vi "observacao_queued.vi"() -> ()   [LabVIEW 2012, in "Shared_160.lvlib"] (continued)
                  tunnel: [TRUE FALSE] -> w2394
                  tunnel: [FALSE TRUE] -> w2393
                  frame False {
                  }
                  frame True {
                  }
                }
                "Recuar" <- w2394
                "Avancar" <- w2393
                n1886 = event shown="[1] \"Sent_EspDesvFeixe\": Value Change" {
                  selector: _ -> [_ _ _]
                  dyn-events: _ -> [_ _ _]
                  timeout: w2396 -> [_ _ _]
                  event Timeout {
                    n1887 = event-data() -> ()  [unwired: 1 in, 2 out]
                  }
                  event "Sent_EspDesvFeixe": Value Change {
                    n1888 = event-data() -> ()  [unwired: 1 in, 4 out]
                    n1889 = case shown="1" "Disabled" {
                      tunnel: ["RECUAR" ("Comando") "AVANCAR" ("Comando")] -> w2443
                      tunnel: ["ESP_LAMP" ("Dispositivo") "ESP_LAMP" ("Dispositivo")] -> w2442
                      frame 0, Default {
                        # "Case False (Default) em\noperação normal, com o\nbotão Sent_EspDesvFeixe\nligado ao ? deste case."
                      }
                      frame 1 {
                        # "CaseTrue. Cf. nota no case 0"
                        n1890 = property on="SlideCam1" class="Slide (strict)"("Visible"=TRUE) -> ()  [unwired: 2 in, 2 out]
                        n1891 = property on="stopCam1" class="Bool"("Visible"=FALSE) -> ()  [unwired: 2 in, 2 out]
                        "SlideCam1" <- u8 5 ("Slide 2")
                      }
                    }
                    n1892 = case shown="True" "Case Constant\n(See Context Help) 9" {
                      tunnel: w2443 -> [_ w2446]
                      tunnel: w2442 -> [_ w2445]
                      frame False {
                      }
                      frame True {
                        w2444 = u16 3 items=["ZERO", "AH", "DEC", "TUBO", "CUP"] ("Controlador")
                        n1893 = call "Monta Comando.vi"("Comando"=w2446, "Dispositivo"=w2445, "Controlador"=w2444) -> ()  [unwired: 4 in, 3 out]
                      }
                    }
                  }
                  event "Go_filtro": Value Change {
                    n1894 = event-data() -> ()  [unwired: 1 in, 6 out]
                    n1895 = case shown="True" "Go_filtro" {
                      frame False {
                      }
                      frame True {
                        (unwired) "ZERO: Porta serial da CAM1"
                        w2455 = u16 0 items=["ZERO", "AH", "DEC", "TUBO", "CUP"] ("Controlador")
                        n1896 = call "Monta Comando.vi"("Set Point"="Filtro", "Controlador"=w2455) -> ()  [unwired: 5 in, 3 out]
                      }
                    }
                  }
                }
                n1897 = case shown="False" "Velocidade" {
                  tunnel: [TRUE FALSE] -> w2391
                  tunnel: [FALSE TRUE] -> w2390
                  frame False {
                  }
                  frame True {
                  }
                }
                "Rapido" <- w2391
                "Lento" <- w2390
                n1898 = call "Bit Status TUBO.vi"("NomeStatus"=w2405) -> ("StatBit"=w2402:bool)
                n1899 = call "Bit Status TUBO.vi"("NomeStatus"=w2404) -> ("StatBit"=w2401:bool)
                n1900 = call "Bit Status TUBO.vi"("NomeStatus"=w2403) -> ("StatBit"=w2400:bool)
                n1901 = Not(x=w2402) -> (.not. x?=w2411:bool)
                n1902 = And(x=w2402, y=w2401) -> (x .and. y?=w2407:bool)
                "LedRepCam1" <- w2407
                n1903 = Or(x=w2401, y=w2400) -> (x .or. y?=w2412:bool)
                n1904 = And(x=w2402, y=w2400) -> (x .and. y?=w2406:bool)
                "LedCalCam1" <- w2406
                n1905 = property on="SlideCam1" class="Slide (strict)"() -> ("Visible"=w2409:bool)  [unwired: 2 in, 2 out]
                n1906 = Or(x=w2407, y=w2406) -> (x .or. y?=w2410:bool)
                n1907 = And(x=w2411, y=w2412) -> (x .and. y?=w2398:bool)
                n1908 = case shown="True" "Case Constant\n(See Context Help) 10" {
                  frame False {
                  }
                  frame True {
                    w2470 = FALSE
                    w2473 = u16 3 items=["ZERO", "AH", "DEC", "TUBO", "CUP"] ("Controlador")
                    w2471 = u8 0 ("Disabled")
                    n1909 = call "Monta Comando.vi"("Comando"="DESLIGAR", "Dispositivo"="ESP_LAMP", "Controlador"=w2473) -> ()  [unwired: 4 in, 3 out]
                    n1910 = property on="Sent_EspDesvFeixe" class="Bool (strict)"("Disabled"=w2471) -> ()  [unwired: 2 in, 2 out]
                    n1911 = property on="Go_filtro" class="Bool"("Disabled"=w2471) -> ()  [unwired: 2 in, 2 out]
                    n1912 = property on="stopCam1" class="Bool"("Visible"=w2470) -> ()  [unwired: 2 in, 2 out]
                    n1913 = property on="SlideCam1" class="Slide (strict)"("Visible"=w2470) -> ()  [unwired: 2 in, 2 out]
                  }
                }
                n1914 = And(x="Case Constant\n(See Context Help) 10", y=w2398) -> (x .and. y?=w2399:bool)
                n1915 = And(x=w2409, y=w2410) -> (x .and. y?=w2408:bool)
                n1916 = case shown="True" w2399 {
                  frame False {
                  }
                  frame True {
                    w2458 = u8 2 ("Disabled")
                    n1917 = local read "SlideCam1"() -> (w2457:u8)
                    n1918 = Add(x=w2457, y=u8 5) -> (x+y=w2459:u8)
                    n1919 = property on="Sent_EspDesvFeixe" class="Bool (strict)"("Disabled"=w2458) -> ()  [unwired: 2 in, 2 out]
                    n1920 = property on="Go_filtro" class="Bool"("Disabled"=w2458) -> ()  [unwired: 2 in, 2 out]
                    n1921 = Greater Or Equal?(x=w2459, y=u8 100 ("x")) -> (x >= y?=w2461:bool)
                    n1922 = case shown="True" w2461 {
                      selector: w2461 -> [_ w2465]
                      tunnel: w2459 -> [w2463 _]
                      frame False {
                        n1923 = local write "SlideCam1"(w2463) -> ()
                        n1924 = property on="SlideCam1" class="Slide (strict)"("Fill Color"=u32 16750950 ("color(black)")) -> ()  [unwired: 2 in, 2 out]
                      }
                      frame True {
                        n1925 = property on="stopCam1" class="Bool"("Visible"=w2465) -> ()  [unwired: 2 in, 2 out]
                        n1926 = local write "SlideCam1"(u8 90 ("Slide 2")) -> ()
                        n1927 = property on="SlideCam1" class="Slide (strict)"("Fill Color"=u32 16724787 ("color(black)")) -> ()  [unwired: 2 in, 2 out]
                      }
                    }
                  }
                }
                n1928 = case shown="True" w2408 {
                  frame False {
                  }
                  frame True {
                    w2469 = u8 0 ("Disabled")
                    n1929 = property on="Go_filtro" class="Bool"("Disabled"=w2469) -> ()  [unwired: 2 in, 2 out]
                    n1930 = property on="Sent_EspDesvFeixe" class="Bool (strict)"("Disabled"=w2469) -> ()  [unwired: 2 in, 2 out]
                    n1931 = property on="SlideCam1" class="Slide (strict)"("Visible"=FALSE) -> ()  [unwired: 2 in, 2 out]
                  }
                }
              }
              frame "Cam 2" {
                # "Cam 2"
              }
              frame "Cam IV." {
                # "Cam IV"
              }
              frame "Polarim." {
                # "Polarimetro"
              }
              frame "Fotrap" {
                # "Fotrap"
              }
              frame "Coude", Default {
                # "COUDE"
                n1932 = stacked-sequence {
                  frame #0 {
                    w2477 = u16 5 items=["Alarme", "Atencao", "Erro", "Ocupado", "Stop#3", "Cass#3", "MovFoco", "PosSecund", "Mov#2", "Mov#3", "Mov#4", "EspLamp", "HE", "NE", "EspLampRepouso", "EspLampCalibra"] ("NomeStatus")
                    w2476 = u16 7 items=["Alarme", "Atencao", "Erro", "Ocupado", "Stop#3", "Cass#3", "MovFoco", "PosSecund", "Mov#2", "Mov#3", "Mov#4", "EspLamp", "HE", "NE", "EspLampRepouso", "EspLampCalibra"] ("NomeStatus")
                    n1933 = local read "EspAtual"() -> (w2479:string)
                    n1934 = case shown="\"A\"" w2479 {
                      frame "X", Default {
                        w2480 = FALSE
                        n1935 = local write "ledVisivel"(w2480) -> ()
                        n1936 = local write "ledAzul"(w2480) -> ()
                        n1937 = local write "ledVermelho"(w2480) -> ()
                      }
                      frame "M" {
                        w2481 = FALSE
                        n1938 = local write "ledAzul"(w2481) -> ()
                        n1939 = local write "ledVermelho"(w2481) -> ()
                        n1940 = local write "ledVisivel"(w2481) -> ()
                      }
                      frame "A" {
                        # "Espelho A --> Azul\nEspelho B --> Visível\nEspelho C --> Vermelho"
                        n1941 = local write "ledVermelho"(FALSE) -> ()
                        n1942 = local write "ledVisivel"(FALSE) -> ()
                        n1943 = local write "ledAzul"(TRUE) -> ()
                      }
                      frame "B" {
                        # "Espelho A --> Azul\nEspelho B --> Visível\nEspelho C --> Vermelho"
                        n1944 = local write "ledVermelho"(FALSE) -> ()
                        n1945 = local write "ledVisivel"(TRUE) -> ()
                        n1946 = local write "ledAzul"(FALSE) -> ()
                      }
                      frame "C" {
                        # "Espelho A --> Azul\nEspelho B --> Visível\nEspelho C --> Vermelho"
                        n1947 = local write "ledVermelho"(TRUE) -> ()
                        n1948 = local write "ledVisivel"(FALSE) -> ()
                        n1949 = local write "ledAzul"(FALSE) -> ()
                      }
                    }
                    n1950 = call "Bit Status TUBO.vi"("NomeStatus"=w2477) -> ("StatBit"=→"Cjto_3":bool)
                    n1951 = call "Bit Status TUBO.vi"("NomeStatus"=w2476) -> ("StatBit"=→"PosSecundario":bool)
                  }
                  frame #1 {
                    w2501 = u16 5 items=["Alarme", "Atencao", "Erro", "Ocupado", "Stop#3", "Cass#3", "MovFoco", "PosSecund", "Mov#2", "Mov#3", "Mov#4", "EspLamp", "HE", "NE", "EspLampRepouso", "EspLampCalibra"] ("NomeStatus")
                    w2506 = u16 8 items=["Alarme", "Atencao", "Erro", "Ocupado", "Stop#3", "Cass#3", "MovFoco", "PosSecund", "Mov#2", "Mov#3", "Mov#4", "EspLamp", "HE", "NE", "EspLampRepouso", "EspLampCalibra"] ("NomeStatus")
                    w2507 = u16 9 items=["Alarme", "Atencao", "Erro", "Ocupado", "Stop#3", "Cass#3", "MovFoco", "PosSecund", "Mov#2", "Mov#3", "Mov#4", "EspLamp", "HE", "NE", "EspLampRepouso", "EspLampCalibra"] ("NomeStatus")
                    w2508 = u16 10 items=["Alarme", "Atencao", "Erro", "Ocupado", "Stop#3", "Cass#3", "MovFoco", "PosSecund", "Mov#2", "Mov#3", "Mov#4", "EspLamp", "HE", "NE", "EspLampRepouso", "EspLampCalibra"] ("NomeStatus")
                    w2519 = u16 4 items=["Alarme", "Atencao", "Erro", "Ocupado", "Stop#3", "Cass#3", "MovFoco", "PosSecund", "Mov#2", "Mov#3", "Mov#4", "EspLamp", "HE", "NE", "EspLampRepouso", "EspLampCalibra"] ("NomeStatus")
                    w2520 = u16 3 items=["Alarme", "Atencao", "Erro", "Ocupado", "Stop#3", "Cass#3", "MovFoco", "PosSecund", "Mov#2", "Mov#3", "Mov#4", "EspLamp", "HE", "NE", "EspLampRepouso", "EspLampCalibra"] ("NomeStatus")
                    # "CJTO#3 EM \nMOVIMENTO"
                    n1952 = local read "PosSecundario"() -> (w2499:bool)
                    n1953 = call "Bit Status TUBO.vi"("NomeStatus"=w2520) -> ("StatBit"=w2495:bool)
                    n1954 = call "Bit Status TUBO.vi"("NomeStatus"=w2506) -> ("StatBit"=w2512:bool)
                    "#2" <- w2512
                    n1955 = call "Bit Status TUBO.vi"("NomeStatus"=w2507) -> ("StatBit"=w2511:bool)
                    "#3" <- w2511
                    n1956 = call "Bit Status TUBO.vi"("NomeStatus"=w2508) -> ("StatBit"=w2510:bool)
                    "#4" <- w2510
                    n1957 = call "Bit Status TUBO.vi"("NomeStatus"=w2501) -> ("StatBit"=w2498:bool)
                    n1958 = call "Bit Status TUBO.vi"("NomeStatus"=w2519) -> ("StatBit"=w2497:bool)
                    n1959 = Not Equal?(x=w2499, y=w2498) -> (x != y?=w2500:bool)
                    n1960 = Not(x=w2497) -> (.not. x?=w2493:bool)
                    n1961 = And(x=w2500, y=w2497) -> (x .and. y?=w2494:bool)
                    n1962 = Compound Arithmetic op=OR(w2512, w2511, w2510) -> (w2509:bool)
                    n1963 = Compound Arithmetic op=OR(w2494, w2493, w2495) -> (w2496:bool)
                    n1964 = property on="PosSecundario" class="Bool (strict)"("Blinking"=w2494) -> ()  [unwired: 2 in, 2 out]
                    n1965 = property on="Cjto_3" class="Bool (strict)"("Blinking"=w2494) -> ()  [unwired: 2 in, 2 out]
                    n1966 = case shown="True" w2496 {
                      tunnel: [T6."Page Enabled" ("Page Enabled State") T6."Page Disabled" ("Page Enabled State")] -> w2491
                      tunnel: [u8 0 ("Disabled") u8 2 ("Disabled")] -> w2505
                      frame False {
                      }
                      frame True {
                      }
                    }
                    n1967 = property on="MENSAGEM" class="Str"("Visible"=w2493, "Blinking"=w2493) -> ()  [unwired: 2 in, 2 out]
                    n1968 = case shown="True" w2509 {
                      tunnel: w2505 -> [w2524 _]
                      tunnel: [w2524 u8 2 ("Disabled")] -> w2504
                      tunnel: [FALSE TRUE] -> w2503
                      tunnel: [FALSE ("Blinking") TRUE ("Blinking")] -> w2502
                      frame False {
                        n1969 = local write "MENSAGEM 2"("EM MOVIMENTO" ("MENSAGEM 2")) -> ()
                      }
                      frame True {
                        n1970 = local read "EndTime"() -> (w2533:u32)
                        n1971 = Tick Count (ms)() -> (millisecond timer value=w2532:u32)
                        n1972 = Subtract(x=w2533, y=w2532) -> (x-y=w2531:u32)
                        n1973 = Divide(x=w2531, y=u32 1000) -> (x/y=w2528:dbl)
                        n1974 = To Unsigned Long Integer(number=w2528) -> (unsigned 32bit integer=w2529:u32)
                        n1975 = Number To Decimal String(number=w2529) -> (decimal integer string=w2526:string)  [unwired: 1 in]
                        n1976 = Concatenate Strings("EM MOVIMENTO " ("MENSAGEM 2"), w2526) -> (w2527:string)
                        n1977 = local write "MENSAGEM 2"(w2527) -> ()
                      }
                    }
                    n1978 = property on="Setup, Pointing & Guiding" class="TabCtl (strict)"() -> ("Pages"=w2492:refnum<vi>[])  [unwired: 2 in, 2 out]
                    n1979 = Index Array(array=w2492, index=4) -> (element=w2515:refnum<vi>)
                    n1980 = Index Array(array=w2492, index=5) -> (element=w2518:refnum<vi>)
                    n1981 = property class="Page"(reference=w2515, "Page Enabled State"=w2491) -> ()  [unwired: 1 in, 2 out]
                    n1982 = property class="Page"(reference=w2518, "Page Enabled State"=w2491) -> ()  [unwired: 1 in, 2 out]
                    n1983 = case shown="False" w2499 {
                      tunnel: [u8 0 ("Disabled") w2539] -> w2514
                      tunnel: w2504 -> [w2537 _]
                      tunnel: [w2537 w2539] -> w2513
                      frame False {
                        # "COUDE"
                      }
                      frame True {
                        w2539 = u8 2 ("Disabled")
                        # "CASS"
                      }
                    }
                    n1984 = property on="MENSAGEM 2" class="Str"("Visible"=w2503, "Blinking"=w2502) -> ()  [unwired: 2 in, 2 out]
                    n1985 = property on="ledAzul" class="Bool (strict)"("Disabled"=w2514) -> ()  [unwired: 2 in, 2 out]
                    n1986 = property on="ledVisivel" class="Bool (strict)"("Disabled"=w2514) -> ()  [unwired: 2 in, 2 out]
                    n1987 = property on="ledVermelho" class="Bool (strict)"("Disabled"=w2514) -> ()  [unwired: 2 in, 2 out]
                    n1988 = property on="Radio Buttons" class="RadioBtnsControl (strict)"("Disabled"=w2514) -> ()  [unwired: 2 in, 2 out]
                    n1989 = property on="#2" class="Bool (strict)"("Disabled"=w2514) -> ()  [unwired: 2 in, 2 out]
                    n1990 = property on="#3" class="Bool (strict)"("Disabled"=w2514) -> ()  [unwired: 2 in, 2 out]
                    n1991 = property on="#4" class="Bool (strict)"("Disabled"=w2514) -> ()  [unwired: 2 in, 2 out]
                    n1992 = property on="Go_Coudé" class="Bool"("Disabled"=w2513) -> ()  [unwired: 2 in, 2 out]
                  }
                  frame #2 {
                    n1993 = case shown="False" "Go_Coudé" {
                      frame False {
                        w2545 = u16 2 items=["Alarme", "Atencao", "Erro", "Ocupado", "Stop#3", "Cass#3", "MovFoco", "PosSecund", "Mov#2", "Mov#3", "Mov#4", "EspLamp", "HE", "NE", "EspLampRepouso", "EspLampCalibra"] ("NomeStatus")
                        w2546 = u16 3 items=["Alarme", "Atencao", "Erro", "Ocupado", "Stop#3", "Cass#3", "MovFoco", "PosSecund", "Mov#2", "Mov#3", "Mov#4", "EspLamp", "HE", "NE", "EspLampRepouso", "EspLampCalibra"] ("NomeStatus")
                        # "TRATA ERROS DO CONTROLADOR"
                        n1994 = call "Bit Status TUBO.vi"("NomeStatus"=w2545) -> ("StatBit"=w2548:bool)
                        n1995 = call "Bit Status TUBO.vi"("NomeStatus"=w2546) -> ("StatBit"=w2550:bool)
                        n1996 = Not(x=w2550) -> (.not. x?=w2549:bool)
                        n1997 = And(x=w2548, y=w2549) -> (x .and. y?=w2547:bool)
                        n1998 = case shown="True" w2547 {
                          frame False {
                          }
                          frame True {
                            w2553 = u16 3 items=["ZERO", "AH", "DEC", "TUBO", "CUP"] ("Controlador")
                            n1999 = call "Monta Comando.vi"("Comando"="ERROS", "Dispositivo"="PROG" ("Comando"), "Controlador"=w2553) -> ()  [unwired: 4 in, 3 out]
                          }
                        }
                      }
                      frame True {
                        w2554 = u16 3 items=["ZERO", "AH", "DEC", "TUBO", "CUP"] ("Controlador")
                        # "Enviar comando de \nmudar Espelho ABC"
                        n2000 = local read "EspAtual"() -> (w2560:string)
                        n2001 = case shown="\"Visível\"" "Radio Buttons" {
                          tunnel: ["C" ("Comando") "A" ("Comando") "B" ("Comando")] -> w2555
                          tunnel: w2560 -> [w2563 w2569 w2574]
                          tunnel: [w2562 w2568 w2575] -> w2557
                          frame "Vermelho" {
                            n2002 = case shown="\"A\"" w2563 {
                              tunnel: [u32 0 u32 60000 u32 35000] -> w2562
                              frame "C", Default {
                              }
                              frame "B" {
                              }
                              frame "A" {
                              }
                            }
                          }
                          frame "Azul", Default {
                            n2003 = case shown="\"C\"" w2569 {
                              tunnel: [u32 0 u32 35000 u32 60000] -> w2568
                              frame "A", Default {
                              }
                              frame "B" {
                              }
                              frame "C" {
                              }
                            }
                          }
                          frame "Visível" {
                            n2004 = case shown="\"C\"" w2574 {
                              tunnel: [u32 0 u32 60000 u32 35000] -> w2575
                              frame "B", Default {
                              }
                              frame "A" {
                              }
                              frame "C" {
                              }
                            }
                          }
                        }
                        n2005 = Tick Count (ms)() -> (millisecond timer value=w2559:u32)
                        n2006 = Add(x=w2559, y=w2557) -> (x+y=→"EndTime":u32)
                        n2007 = call "Monta Comando.vi"("Comando"=w2555, "Dispositivo"="ESPELHO" ("Comando"), "Controlador"=w2554) -> ()  [unwired: 4 in, 3 out]
                      }
                    }
                  }
                  frame #3 {
                    w2586 = 360.0
                    w2591 = 6.283185307179586
                    n2008 = global read "Global_Telescopio.vi" "guide_ang"() -> (w2601:string)
                    n2009 = global read "Global_Telescopio.vi" "guide_nor"() -> (w2602:string)
                    n2010 = global read "Global_Telescopio.vi" "AH_now"() -> (w2598:dbl)
                    n2011 = global read "Global_Telescopio.vi" "delta_now"() -> (w2599:dbl)
                    n2012 = Add(x=w2598, y=w2599) -> (x+y=w2590:dbl)
                    n2013 = Fract/Exp String To Number(string=w2601) -> (number=w2597:dbl)  [unwired: 3 in, 1 out]
                    n2014 = Fract/Exp String To Number(string=w2602) -> (number=w2600:dbl)  [unwired: 3 in, 1 out]
                    n2015 = Quotient & Remainder(x=w2590, y=w2591) -> (x-y*floor(x/y)=w2593:dbl)  [unwired: 1 out]
                    n2016 = Add(x=w2597, y=w2600) -> (x+y=w2582:dbl)
                    n2017 = Less Than 0?(x=w2593) -> (x < 0?=w2595:bool)
                    n2018 = case shown="True" w2595 {
                      tunnel: w2593 -> [w2603 w2606]
                      tunnel: [w2603 w2604] -> w2592
                      tunnel: w2591 -> [_ w2605]
                      frame False {
                      }
                      frame True {
                        n2019 = Add(x=w2606, y=w2605) -> (x+y=w2604:dbl)
                      }
                    }
                    n2020 = Add(x=124.0, y=w2582) -> (x+y=w2581:dbl)
                    n2021 = Multiply(x=w2592, y=57.29577951 ("x*y")) -> (x*y=w2589:dbl)
                    n2022 = Subtract(x=98.2, y=w2589) -> (x-y=w2588:dbl)
                    n2023 = Add(x=w2581, y=w2588) -> (x+y=w2585:dbl)
                    n2024 = Quotient & Remainder(x=w2585, y=w2586) -> (floor(x/y)=w2587:dbl)  [unwired: 1 out]
                    n2025 = Multiply(x=w2587, y=w2586) -> (x*y=w2584:dbl)
                    n2026 = Subtract(x=w2585, y=w2584) -> (x-y=→"Ang. Fenda":dbl)
                  }
                  frame #4 {
                    # "90"
                    # "270"
                    # "180"
                    # "0"
                    n2027 = event shown="[0] Timeout" {
                      selector: _ -> [_ _ _ _ _ _ _ _ _ _ _]
                      dyn-events: _ -> [_ _ _ _ _ _ _ _ _ _ _]
                      timeout: 10 -> [_ _ _ _ _ _ _ _ _ _ _]
                      event Timeout {
                        n2028 = event-data() -> ()  [unwired: 1 in, 2 out]
                        n2029 = stacked-sequence {
                          frame #0 {
                            n2030 = local read "parou 3"() -> (w2608:bool)
                            n2031 = case shown="True" w2608 {
                              frame False {
                              }
                              frame True {
                                n2032 = call "InstrumentControl.vi"("Input Message"="COUDE REDE POSICAO") -> ("Output Message"=w2611:string)  [unwired: 9 in, 1 out]
                                "Output Message" <- w2611
                                n2033 = Decimal String To Number(string=w2611) -> (number=w2610:i32)  [unwired: 2 in, 1 out]
                                n2034 = while {
                                shift-right: [w2614] -> w2609
                                shift-left: _ -> [w2618]
                                tunnel: w2610 -> [w2614]
                                stop <- TRUE stop-if-true
                                n2035 = Subtract(x=w2618, y=w2614) -> (x-y=w2617:i32)
                                n2036 = Absolute Value(x=w2617) -> (abs(x)=w2616:i32)
                                n2037 = Greater Or Equal?(x=w2616, y=1) -> (x >= y?=→"parou 3":bool)
                                }
                                "Posição Rede" <- w2609
                              }
                            }
                          }
                          frame #1 {
                            n2038 = local read "parou"() -> (w2621:bool)
                            n2039 = local read "parou 2"() -> (w2620:bool)
                            n2040 = case shown="True" w2620 {
                              frame False {
                              }
                              frame True {
                                # "Cada volta -> 10mm\nCada volta -> 4000counts\n1 count = 0,0025mm"
                                n2041 = call "InstrumentControl.vi"("Input Message"="COUDE ESPELHO POSICAO") -> ("Output Message"=w2628:string)  [unwired: 9 in, 1 out]
                                n2042 = Fract/Exp String To Number(string=w2628) -> (number=w2627:dbl)  [unwired: 3 in, 1 out]
                                n2043 = while {
                                shift-right: [w2640] -> w2623
                                shift-left: _ -> [w2641]
                                tunnel: w2627 -> [w2640]
                                tunnel: [w2636] -> w2622
                                stop <- TRUE stop-if-true
                                n2044 = Subtract(x=w2641, y=w2640) -> (x-y=w2639:dbl)
                                n2045 = Absolute Value(x=w2639) -> (abs(x)=w2638:dbl)
                                n2046 = Greater Or Equal?(x=w2638, y=0.02) -> (x >= y?=w2636:bool)
                                "parou 2" <- w2636
                                }
                                "Posição Espelho" <- w2623
                                n2047 = case shown="False" w2622 {
                                frame False {
                                n2048 = call "InstrumentControl.vi"("Input Message"="COUDE SERIAL CHAVEAR OFF") -> ()  [unwired: 9 in, 2 out]
                                }
                                frame True {
                                }
                                }
                                n2049 = Absolute Value(x=w2623) -> (abs(x)=w2624:dbl)
                                n2050 = Less Or Equal?(x=w2624, y=0.5) -> (x <= y?=w2626:bool)
                                n2051 = case shown="False" w2626 {
                                tunnel: w2624 -> [w2633 _]
                                frame False {
                                n2052 = Greater Or Equal?(x=w2633, y=34.5) -> (x >= y?=w2631:bool)
                                n2053 = case shown="True" w2631 {
                                frame False {
                                }
                                frame True {
                                n2054 = local write "Boolean"(TRUE ("Boolean")) -> ()
                                }
                                }
                                }
                                frame True {
                                n2055 = local write "Boolean"(FALSE ("Boolean")) -> ()
                                }
                                }
                              }
                            }
                            n2056 = case shown="True" w2621 {
                              frame False {
                              }
                              frame True {
                                n2057 = call "InstrumentControl.vi"("Input Message"="COUDE FENDA POSICAO") -> ("Output Message"=w2648:string)  [unwired: 9 in, 1 out]
                                n2058 = Fract/Exp String To Number(string=w2648) -> (number=w2647:dbl)  [unwired: 3 in, 1 out]
                                n2059 = Multiply(x=w2647, y=1000.0) -> (x*y=w2645:dbl)
                                n2060 = while {
                                shift-right: [w2655] -> w2644
                                shift-left: _ -> [w2656]
                                tunnel: w2645 -> [w2655]
                                tunnel: [w2651] -> w2643
                                stop <- TRUE stop-if-true
                                n2061 = Subtract(x=w2656, y=w2655) -> (x-y=w2654:dbl)
                                n2062 = Absolute Value(x=w2654) -> (abs(x)=w2653:dbl)
                                n2063 = Greater Or Equal?(x=w2653, y=1.0) -> (x >= y?=w2651:bool)
                                "parou" <- w2651
                                }
                                "Largura da Fenda 2" <- w2644
                                n2064 = case shown="False" w2643 {
                                frame False {
                                n2065 = call "InstrumentControl.vi"("Input Message"="COUDE SERIAL CHAVEAR OFF") -> ()  [unwired: 9 in, 2 out]
                                }
                                frame True {
                                }
                                }
                              }
                            }
                          }
                        }
                      }
                      event "Cathode": Value Change {
                        n2066 = event-data() -> ("NewVal"=w2658:bool)  [unwired: 1 in, 4 out]
                        n2067 = case shown="True" w2658 {
                          frame False {
                          }
                          frame True {
                            n2068 = flat-sequence {
                              frame #0 {
                                w2660 = FALSE ("NeAr")
                                n2069 = local write "Neon"(w2660) -> ()
                                n2070 = local write "Incand"(w2660) -> ()
                                n2071 = local write "Position"("Moving" ("Prisma Position")) -> ()
                                n2072 = call "Comando_Quick_Silver.vi"("COMANDO COMPLETO"="COUDE PRISMA MOVER 0" ("Input Message")) -> ()  [unwired: 2 in, 3 out]
                                n2073 = local write "IronArc"(w2660) -> ()
                              }
                              frame #1 {
                                n2074 = Wait (ms)(milliseconds to wait=u32 50) -> ()  [unwired: 1 out]
                              }
                              frame #2 {
                                n2075 = local write "Position"("Cathode" ("Prisma Position")) -> ()
                              }
                            }
                          }
                        }
                      }
                      event "Neon": Value Change {
                        n2076 = event-data() -> ("NewVal"=w2664:bool)  [unwired: 1 in, 4 out]
                        n2077 = case shown="True" w2664 {
                          frame False {
                          }
                          frame True {
                            n2078 = flat-sequence {
                              frame #0 {
                                w2666 = FALSE ("ThAr")
                                n2079 = local write "Cathode"(w2666) -> ()
                                n2080 = local write "Incand"(w2666) -> ()
                                n2081 = local write "Position"("Moving" ("Prisma Position")) -> ()
                                n2082 = call "Comando_Quick_Silver.vi"("COMANDO COMPLETO"="COUDE PRISMA MOVER 180" ("Input Message")) -> ()  [unwired: 2 in, 3 out]
                                n2083 = local write "IronArc"(w2666) -> ()
                              }
                              frame #1 {
                                n2084 = Wait (ms)(milliseconds to wait=u32 50) -> ()  [unwired: 1 out]
                              }
                              frame #2 {
                                n2085 = local write "Position"("Neon" ("Prisma Position")) -> ()
                              }
                            }
                          }
                        }
                      }
                      event "Incand": Value Change {
                        n2086 = event-data() -> ("NewVal"=w2670:bool)  [unwired: 1 in, 4 out]
                        n2087 = case shown="True" w2670 {
                          frame False {
                          }
                          frame True {
                            n2088 = flat-sequence {
                              frame #0 {
                                w2672 = FALSE ("ThAr")
                                n2089 = local write "Cathode"(w2672) -> ()
                                n2090 = local write "Neon"(w2672) -> ()
                                n2091 = local write "Position"("Moving" ("Prisma Position")) -> ()
                                n2092 = call "Comando_Quick_Silver.vi"("COMANDO COMPLETO"="COUDE PRISMA MOVER 270 " ("Input Message")) -> ()  [unwired: 2 in, 3 out]
                                n2093 = local write "IronArc"(w2672) -> ()
                              }
                              frame #1 {
                                n2094 = Wait (ms)(milliseconds to wait=u32 50) -> ()  [unwired: 1 out]
                              }
                              frame #2 {
                                n2095 = local write "Position"("Incand" ("Prisma Position")) -> ()
                              }
                            }
                          }
                        }
                      }
                      event Value Change {
                        n2096 = event-data() -> ("NewVal"=w2676:T4)  [unwired: 1 in, 4 out]
                        n2097 = case shown="True" w2676 {
                          frame False {
                          }
                          frame True {
                            n2098 = call "InstrumentControl.vi"("Input Message"="COUDE FENDA INICIAR") -> ()  [unwired: 9 in, 2 out]
                          }
                        }
                      }
                      event Value Change {
                        n2099 = event-data() -> ("NewVal"=w2678:T4)  [unwired: 1 in, 4 out]
                        n2100 = case shown="True" w2678 {
                          frame False {
                          }
                          frame True {
                            n2101 = call "Comando_Quick_Silver.vi"("COMANDO COMPLETO"="COUDE ESPELHO INICIAR" ("Input Message")) -> ()  [unwired: 2 in, 3 out]
                          }
                        }
                      }
                      event Value Change {
                        n2102 = event-data() -> ("NewVal"=w2680:T4)  [unwired: 1 in, 4 out]
                        n2103 = case shown="True" w2680 {
                          frame False {
                          }
                          frame True {
                            n2104 = call "InstrumentControl.vi"("Input Message"="COUDE PRISMA INICIAR") -> ()  [unwired: 9 in, 2 out]
                          }
                        }
                      }
                      event "Go Angulo de Difração": Value Change {
                        n2105 = event-data() -> ("NewVal"=w2682:bool)  [unwired: 1 in, 4 out]
                        n2106 = case shown="True" w2682 {
                          frame False {
                          }
                          frame True {
                            # "Envia comando para rede de difração"
                            n2107 = Number To Decimal String(number="Angulo da rede de difração") -> (decimal integer string=w2684:string)  [unwired: 1 in]
                            n2108 = Concatenate Strings("COUDE REDE MOVER ", w2684) -> (w2687:string)
                            n2109 = call "InstrumentControl.vi"("Input Message"=w2687) -> ()  [unwired: 9 in, 2 out]
                            n2110 = local write "parou 3"(TRUE ("parou 3")) -> ()
                          }
                        }
                      }
                      event "Go Largura da Fenda": Value Change {
                        n2111 = event-data() -> ("NewVal"=w2688:bool)  [unwired: 1 in, 4 out]
                        n2112 = case shown="True" w2688 {
                          frame False {
                          }
                          frame True {
                            n2113 = call "InstrumentControl.vi"("Input Message"="COUDE SERIAL CHAVEAR ON") -> ("error out"=w2690:errorcluster)  [unwired: 9 in, 1 out]
                            n2114 = Divide(x="Largura da Fenda", y=1000.0) -> (x/y=w2698:dbl)
                            n2115 = Number To Fractional String(use system decimal point (T)=FALSE, number=w2698, precision (6)=i16 6) -> (F-format string=w2692:string)  [unwired: 1 in]
                            n2116 = Concatenate Strings("COUDE FENDA MOVER ", w2692) -> (w2694:string)
                            n2117 = local write "parou"(TRUE ("parou")) -> ()
                            n2118 = call "InstrumentControl.vi"("error"=w2690, "Input Message"=w2694) -> ()  [unwired: 8 in, 2 out]
                          }
                        }
                      }
                      event "Prisma das Lâmpadas": Value Change {
                        n2119 = event-data() -> ("NewVal"=w2709:bool)  [unwired: 1 in, 4 out]
                        n2120 = case shown="False" w2709 {
                          tunnel: [0.0 ("y") 35.0 ("y")] -> w2707
                          frame False {
                            n2121 = local write "Boolean"(TRUE ("Boolean")) -> ()
                          }
                          frame True {
                            n2122 = local write "Boolean"(FALSE ("Boolean 2")) -> ()
                          }
                        }
                        n2123 = call "InstrumentControl.vi"("Input Message"="COUDE SERIAL CHAVEAR ON") -> ("error out"=w2701:errorcluster)  [unwired: 9 in, 1 out]
                        n2124 = local write "parou 2"(TRUE ("parou 2")) -> ()
                        n2125 = Number To Fractional String(use system decimal point (T)=FALSE, number=w2707, precision (6)=i16 6) -> (F-format string=w2702:string)  [unwired: 1 in]
                        n2126 = Concatenate Strings("COUDE ESPELHO MOVER ", w2702) -> (w2704:string)
                        n2127 = call "InstrumentControl.vi"("error"=w2701, "Input Message"=w2704) -> ()  [unwired: 8 in, 2 out]
                      }
                      event "IronArc": Value Change {
                        n2128 = event-data() -> ("NewVal"=w2714:bool)  [unwired: 1 in, 4 out]
                        n2129 = case shown="True" w2714 {
                          frame False {
                          }
                          frame True {
                            n2130 = flat-sequence {
                              frame #0 {
                                w2716 = FALSE ("ThAr")
                                n2131 = local write "Cathode"(w2716) -> ()
                                n2132 = local write "Neon"(w2716) -> ()
                                n2133 = local write "Position"("Moving" ("Prisma Position")) -> ()
                                n2134 = call "Comando_Quick_Silver.vi"("COMANDO COMPLETO"="COUDE PRISMA MOVER 90 " ("Input Message")) -> ()  [unwired: 2 in, 3 out]
                                n2135 = local write "Incand"(w2716) -> ()
                              }
                              frame #1 {
                                n2136 = Wait (ms)(milliseconds to wait=u32 50) -> ()  [unwired: 1 out]
                              }
                              frame #2 {
                                n2137 = local write "Position"("IronArc" ("Prisma Position")) -> ()
                              }
                            }
                          }
                        }
                      }
                    }
                  }
                }
              }
            }
          }
          frame "FOCUS" {
            w2743 = cluster{u32, u32}[] [] ("Colors [4]")
            w2744 = cluster{u32, u32}[] [] ("Colors [4]")
            # "ATUALIZA FOCO COM VALORES\nPUBLICADOS PELO FOCUSER160"
            # "dark(0)/bright(1)\n green"
            # "red(0)/greem(1)"
            # "ZeroMQ"
            # "T:  0x54      84\nC: 0x43       51\nS:  0x53      83\nP:  0x50      80\nD:  0x44      52\nClientId= 350"
            n2138 = global read "Global_Telescopio.vi" "queueSUB"() -> (w2738:refnum<queue>)
            n2139 = global read "Global_Telescopio.vi" "Focuser160"() -> (w2734:T11)
            n2140 = Get Queue Status(queue=w2738) -> (queue out=w2735:refnum<queue>, # elements in queue=w2737:i32)  [unwired: 2 in, 6 out]
            n2141 = Greater Than 0?(x=w2737) -> (x > 0?=w2736:bool)
            n2142 = call "TX focus FOCO.vi"("Comando"="pos") -> ("pos (deg)"=→"old":dbl)  [unwired: 12 in, 2 out]
            n2143 = case shown="True" w2736 {
              tunnel: w2735 -> [_ w2794]
              tunnel: w2734 -> [w2785 w2792]
              tunnel: [w2785 w2791] -> w2733
              frame False {
              }
              frame True {
                n2144 = Flush Queue(queue=w2794) -> (remaining elements=w2788:string[], error out=w2793:errorcluster)  [unwired: 1 in, 1 out]
                n2145 = Array Size(array=w2788) -> (size(s)=w2790:i32)
                "size(s)" <- w2790
                n2146 = Decrement(x=w2790) -> (x-1=w2789:i32)
                n2147 = Index Array(array=w2788, index=w2789) -> (element=w2787:string)
                "element" <- w2787
                n2148 = call "Focuser JSON to cluster.vi"("JSON status"=w2787) -> ("Focuser160"=w2786:T11)  [unwired: 10 in]
                n2149 = Select(t=w2792, s=w2793, f=w2786) -> (s? t:f=w2791:T11)
                n2150 = global write "Global_Telescopio.vi" "Focuser160"(w2791) -> ()
              }
            }
            n2151 = Unbundle By Name(w2733) -> ("alarm"=→"focuAlarm":bool, "cmd"=w2731:T12, "connected"=w2730:bool, "maxSpeed"=w2729:dbl, "maxStep"=w2728:dbl, "position"=→"Foco":dbl, "error"=w2723:string, "homing"=→"focusHoming":bool, "initialized"=→"focusInitialized":bool, "isMoving"=→"focusMoving":bool)
            "focusConnected" <- w2730
            n2152 = property on="Foco" class="Slide (strict)"() -> ("Scale.Maximum"=w2768:dbl)  [unwired: 2 in, 2 out]
            n2153 = Unbundle By Name(w2731) -> ("clientId"=w2761:dbl)
            n2154 = Search and Replace String(replace all?=TRUE ("replace all? (F)"), input string=w2723, search string="\"") -> (result string=w2720:string)  [unwired: 5 in, 3 out]
            n2155 = Select(t=w2744, s=w2730, f=w2743) -> (s? t:f=w2741:cluster{u32, u32}[])
            n2156 = Select(t=w2744, s=w2730, f=w2743) -> (s? t:f=w2742:cluster{u32, u32}[])
            n2157 = property on="focusInitialized" class="Bool (strict)"("Colors [4]"=w2741) -> ()  [unwired: 2 in, 2 out]
            n2158 = property on="focuAlarm" class="Bool (strict)"("Colors [4]"=w2742) -> ()  [unwired: 2 in, 2 out]
            n2159 = case shown="True" "SetDefaultFocus" {
              frame False {
              }
              frame True {
                n2160 = global read "Global_Telescopio.vi" "Foco Instrumento"() -> (w2855:string)
                n2161 = Fract/Exp String To Number(string=w2855) -> (number=w2854:dbl)  [unwired: 3 in, 1 out]
                n2162 = local write "Setpoint"(w2854) -> ()
              }
            }
            n2163 = disable-structure shown="Disabled" {
              disable-tunnel: 350.0 ("x") -> [w2784 _]
              disable-tunnel: w2761 -> [w2783 _]
              disable-tunnel: w2730 -> [w2770 _]
              frame Disabled {
                w2771 = T5."Disabled and Grayed Out" ("Disabled")
                w2772 = T5."Enabled" ("Disabled")
                n2164 = property on="GO" class="Bool"() -> ("BoolText.Text"=w2776:string)  [unwired: 2 in, 2 out]
                n2165 = Not Equal?(x=w2784, y=w2783) -> (x != y?=w2780:bool)
                n2166 = Not Equal To 0?(x=w2783) -> (x != 0?=w2779:bool)
                n2167 = Not(x=w2770) -> (.not. x?=w2777:bool)
                n2168 = And(x=w2780, y=w2779) -> (x .and. y?=w2781:bool)
                n2169 = Or(x=w2781, y=w2777) -> (x .or. y?=w2778:bool)
                n2170 = Equal?(x=w2776, y="STOP" ("controller")) -> (x = y?=w2773:bool)
                n2171 = Select(t=w2771, s=w2778, f=w2772) -> (s? t:f=w2782:T5)
                n2172 = Select(t=w2771, s=w2773, f=w2772) -> (s? t:f=w2774:T5)
                n2173 = property on="GO" class="Bool"("Disabled"=w2782) -> ()  [unwired: 2 in, 2 out]
                n2174 = property on="focusHome" class="Bool"("DisabledEnum"=w2782) -> ()  [unwired: 2 in, 2 out]
                n2175 = property on="Focus -" class="Bool (strict)"("Disabled"=w2782) -> ()  [unwired: 2 in, 2 out]
                n2176 = property on="Focus +" class="Bool (strict)"("Disabled"=w2782) -> ()  [unwired: 2 in, 2 out]
                n2177 = property on="focusHome" class="Bool"("DisabledEnum"=w2774) -> ()  [unwired: 2 in, 2 out]
                n2178 = property on="Focus -" class="Bool (strict)"("Disabled"=w2774) -> ()  [unwired: 2 in, 2 out]
                n2179 = property on="Focus +" class="Bool (strict)"("Disabled"=w2774) -> ()  [unwired: 2 in, 2 out]
              }
              frame Enabled {
              }
            }
            n2180 = Multiply(x=w2729, y="Velocity") -> (x*y=w2750:dbl)
            n2181 = Greater Than 0?(x=w2728) -> (x > 0?=w2766:bool)
            n2182 = Empty String/Path?(string/path=w2720) -> (empty?=w2765:bool)
            n2183 = To Unsigned Word Integer(number=w2729) -> (unsigned 16bit integer=w2760:u16)
            n2184 = Number To Decimal String(number=w2760) -> (decimal integer string=w2758:string)  [unwired: 1 in]
            n2185 = And(x=w2730, y=w2766) -> (x .and. y?=w2752:bool)
            n2186 = Number To Fractional String(number=w2750, precision (6)=i16 2) -> (F-format string=w2745:string)  [unwired: 2 in]
            n2187 = Concatenate Strings("(max = " ("string"), w2758, " u/s)" ("string")) -> (w2749:string)
            n2188 = Select(t=w2728, s=w2752, f=w2768) -> (s? t:f=w2767:dbl)
            n2189 = Select(t="            Focus Status", s=w2765, f=w2720) -> (s? t:f=→"focusStatus":string)
            n2190 = property on="Foco" class="Slide (strict)"("Scale.Maximum"=w2767) -> ()  [unwired: 2 in, 2 out]
            n2191 = property on="Velocity" class="Slide (strict)"("Caption.Text"=w2749) -> ()  [unwired: 2 in, 2 out]
            n2192 = disable-structure shown="Disabled" {
              frame Disabled {
                n2193 = property on="focusStatus" class="Str" props=["TipStrip"]() -> ()  [unwired: 2 in, 3 out]
              }
              frame Enabled {
              }
            }
            n2194 = property on="Focus -" class="Bool (strict)"() -> ("DisabledEnum"=w2753:T5)  [unwired: 2 in, 2 out]
            n2195 = property on="Focus +" class="Bool (strict)"() -> ("DisabledEnum"=w2746:T5)  [unwired: 2 in, 2 out]
            n2196 = case shown="True" "focusHome" {
              frame False {
              }
              frame True {
                n2197 = property on="GO" class="Bool"("BoolText.Text"="STOP" ("controller")) -> ()  [unwired: 2 in, 2 out]
                n2198 = property on="Foco" class="Slide (strict)"() -> ("Caption.Text"=w2853:string)  [unwired: 2 in, 2 out]
                n2199 = Decimal String To Number(string=w2853) -> (number=w2850:i32)  [unwired: 2 in, 1 out]
                n2200 = Increment(x=w2850) -> (x+1=w2848:i32)
                n2201 = Number To Decimal String(number=w2848) -> (decimal integer string=w2852:string)  [unwired: 1 in]
                n2202 = call "Focus PUSH.vi"("action"="HOME" ("controller"), "clientTransactionId"=w2850) -> ()  [unwired: 9 in, 1 out]
                n2203 = property on="Foco" class="Slide (strict)"("Caption.Text"=w2852) -> ()  [unwired: 2 in, 2 out]
              }
            }
            n2204 = case shown="True" "GO" {
              frame False {
              }
              frame True {
                w2836 = "GO" ("controller")
                n2205 = property on="GO" class="Bool"() -> ("BoolText.Text"=w2846:string)  [unwired: 2 in, 2 out]
                n2206 = property on="Foco" class="Slide (strict)"() -> ("Caption.Text"=w2843:string)  [unwired: 2 in, 2 out]
                n2207 = Equal?(x=w2846, y=w2836) -> (x = y?=w2837:bool)
                n2208 = Number To Decimal String(number="Setpoint") -> (decimal integer string=w2840:string)  [unwired: 1 in]
                n2209 = Decimal String To Number(string=w2843) -> (number=w2845:i32)  [unwired: 2 in, 1 out]
                n2210 = Concatenate Strings("MOVE=" ("controller"), w2840) -> (w2839:string)
                n2211 = Increment(x=w2845) -> (x+1=w2832:i32)
                n2212 = Number To Decimal String(number=w2832) -> (decimal integer string=w2844:string)  [unwired: 1 in]
                n2213 = Select(t=w2839, s=w2837, f="HALT" ("controller")) -> (s? t:f=w2838:string)
                n2214 = Select(t="STOP" ("controller"), s=w2837, f=w2836) -> (s? t:f=w2835:string)
                n2215 = property on="Foco" class="Slide (strict)"("Caption.Text"=w2844) -> ()  [unwired: 2 in, 2 out]
                n2216 = call "Focus PUSH.vi"("action"=w2838, "clientTransactionId"=w2845) -> ()  [unwired: 9 in, 1 out]
                n2217 = disable-structure shown="Disabled" {
                  disable-tunnel: w2835 -> [w2847 _]
                  frame Disabled {
                    n2218 = property on="GO" class="Bool"("BoolText.Text"=w2847) -> ()  [unwired: 2 in, 2 out]
                  }
                  frame Enabled {
                  }
                }
              }
            }
            n2219 = case shown="True" "Focus +" {
              tunnel: w2753 -> [w2814 w2825]
              tunnel: w2745 -> [w2813 w2824]
              frame True {
                n2220 = case shown="\"Enabled\"" w2814 {
                  tunnel: w2813 -> [w2819 _]
                  frame "Enabled" {
                    w2815 = T5."Disabled" ("Disabled")
                    n2221 = property on="Foco" class="Slide (strict)"() -> ("Caption.Text"=w2821:string)  [unwired: 2 in, 2 out]
                    n2222 = Decimal String To Number(string=w2821) -> (number=w2823:i32)  [unwired: 2 in, 1 out]
                    n2223 = Concatenate Strings("FOCUSOUT=" ("controller"), w2819) -> (w2818:string)
                    n2224 = property on="Focus -" class="Bool (strict)"("DisabledEnum"=T5."Disabled" ("Disabled")) -> ()  [unwired: 2 in, 2 out]
                    n2225 = Increment(x=w2823) -> (x+1=w2816:i32)
                    n2226 = Number To Decimal String(number=w2816) -> (decimal integer string=w2822:string)  [unwired: 1 in]
                    n2227 = call "Focus PUSH.vi"("action"=w2818, "clientTransactionId"=w2823) -> ()  [unwired: 9 in, 1 out]
                    n2228 = property on="Foco" class="Slide (strict)"("Caption.Text"=w2822) -> ()  [unwired: 2 in, 2 out]
                    n2229 = property on="GO" class="Bool"("DisabledEnum"=w2815) -> ()  [unwired: 2 in, 2 out]
                    n2230 = property on="focusHome" class="Bool"("DisabledEnum"=w2815) -> ()  [unwired: 2 in, 2 out]
                  }
                  frame "Disabled", Default {
                  }
                }
              }
              frame False {
                n2231 = case shown="\"Disabled\"" w2825 {
                  tunnel: w2824 -> [_ _]
                  frame "Disabled" {
                    w2827 = T5."Enabled" ("Disabled")
                    n2232 = property on="Foco" class="Slide (strict)"() -> ("Caption.Text"=w2829:string)  [unwired: 2 in, 2 out]
                    n2233 = Decimal String To Number(string=w2829) -> (number=w2831:i32)  [unwired: 2 in, 1 out]
                    n2234 = Increment(x=w2831) -> (x+1=w2826:i32)
                    n2235 = Number To Decimal String(number=w2826) -> (decimal integer string=w2830:string)  [unwired: 1 in]
                    n2236 = call "Focus PUSH.vi"("action"="HALT" ("controller"), "clientTransactionId"=w2831) -> ()  [unwired: 9 in, 1 out]
                    n2237 = property on="Foco" class="Slide (strict)"("Caption.Text"=w2830) -> ()  [unwired: 2 in, 2 out]
                    n2238 = property on="Focus -" class="Bool (strict)"("DisabledEnum"=w2827) -> ()  [unwired: 2 in, 2 out]
                    n2239 = property on="GO" class="Bool"("DisabledEnum"=w2827) -> ()  [unwired: 2 in, 2 out]
                    n2240 = property on="focusHome" class="Bool"("DisabledEnum"=w2827) -> ()  [unwired: 2 in, 2 out]
                  }
                  frame "Enabled", Default {
                  }
                }
              }
            }
            n2241 = case shown="False" "Focus -" {
              tunnel: w2746 -> [w2796 w2806]
              tunnel: w2745 -> [w2795 w2805]
              frame True {
                n2242 = case shown="\"Enabled\"" w2796 {
                  tunnel: w2795 -> [_ w2800]
                  frame "Disabled", Default {
                  }
                  frame "Enabled" {
                    w2798 = T5."Disabled" ("Disabled")
                    n2243 = property on="Foco" class="Slide (strict)"() -> ("Caption.Text"=w2802:string)  [unwired: 2 in, 2 out]
                    n2244 = Decimal String To Number(string=w2802) -> (number=w2804:i32)  [unwired: 2 in, 1 out]
                    n2245 = Concatenate Strings("FOCUSIN=" ("controller"), w2800) -> (w2799:string)
                    n2246 = Increment(x=w2804) -> (x+1=w2797:i32)
                    n2247 = Number To Decimal String(number=w2797) -> (decimal integer string=w2803:string)  [unwired: 1 in]
                    n2248 = call "Focus PUSH.vi"("action"=w2799, "clientTransactionId"=w2804) -> ()  [unwired: 9 in, 1 out]
                    n2249 = property on="Foco" class="Slide (strict)"("Caption.Text"=w2803) -> ()  [unwired: 2 in, 2 out]
                    n2250 = property on="Focus +" class="Bool (strict)"("DisabledEnum"=w2798) -> ()  [unwired: 2 in, 2 out]
                    n2251 = property on="GO" class="Bool"("DisabledEnum"=w2798) -> ()  [unwired: 2 in, 2 out]
                    n2252 = property on="focusHome" class="Bool"("DisabledEnum"=w2798) -> ()  [unwired: 2 in, 2 out]
                  }
                }
              }
              frame False {
                n2253 = case shown="\"Disabled\"" w2806 {
                  tunnel: w2805 -> [_ _]
                  frame "Disabled" {
                    w2808 = T5."Enabled" ("Disabled")
                    n2254 = property on="Foco" class="Slide (strict)"() -> ("Caption.Text"=w2810:string)  [unwired: 2 in, 2 out]
                    n2255 = Decimal String To Number(string=w2810) -> (number=w2812:i32)  [unwired: 2 in, 1 out]
                    n2256 = Increment(x=w2812) -> (x+1=w2807:i32)
                    n2257 = Number To Decimal String(number=w2807) -> (decimal integer string=w2811:string)  [unwired: 1 in]
                    n2258 = call "Focus PUSH.vi"("action"="HALT" ("controller"), "clientTransactionId"=w2812) -> ()  [unwired: 9 in, 1 out]
                    n2259 = property on="Foco" class="Slide (strict)"("Caption.Text"=w2811) -> ()  [unwired: 2 in, 2 out]
                    n2260 = property on="Focus +" class="Bool (strict)"("DisabledEnum"=w2808) -> ()  [unwired: 2 in, 2 out]
                    n2261 = property on="GO" class="Bool"("DisabledEnum"=w2808) -> ()  [unwired: 2 in, 2 out]
                    n2262 = property on="focusHome" class="Bool"("DisabledEnum"=w2808) -> ()  [unwired: 2 in, 2 out]
                  }
                  frame "Enabled", Default {
                  }
                }
              }
            }
          }
          frame "ROTATOR" {
            # "MUDANÇA 22/6/11:\nValor default passou a ser carregado no início deste VI."
            n2263 = local read "Default Angle"() -> (w2858:string)
            n2264 = global read "Global_Telescopio.vi" "rotator_def"() -> (w2859:string)
            n2265 = Not Equal?(x=w2859, y=w2858) -> (x != y?=w2857:bool)
            n2266 = case shown="True" "Set Rotator Angle" {
              frame False {
              }
              frame True {
                # "MUDANÇA 22/6/11:\nIncluída a formatação\nda string"
                n2267 = call "Formata_Numeros.vi"("Formato ex-> 7.2"="7.2", "Valor num"="New Angle") -> ("resulting string"=w2865:string)
                "Rotator Angle" <- w2865
                n2268 = global write "Global_Telescopio.vi" "guide_ang"(w2865) -> ()
              }
            }
            n2269 = global write "Global_Telescopio.vi" "Flag-Rotator"(FALSE ("Flag-Rotator")) -> ()
            n2270 = case shown="True" "SetRotatorDefAngle" {
              tunnel: w2858 -> [_ w2863]
              frame False {
              }
              frame True {
                n2271 = local write "Rotator Angle"(w2863) -> ()
                n2272 = global write "Global_Telescopio.vi" "guide_ang"(w2863) -> ()
              }
            }
            n2273 = case shown="True" w2857 {
              tunnel: w2859 -> [_ w2862]
              frame False {
              }
              frame True {
                n2274 = local write "Rotator Angle"(w2862) -> ()
                n2275 = global write "Global_Telescopio.vi" "guide_ang"(w2862) -> ()
                "Default Angle" <- w2862
              }
            }
          }
          frame "DOME" {
            w2880 = u16 6 items=["Alarme", "Atencao", "Erro", "Ocupado", "TBD", "LCB", "Trapeira", "Paravento", "DomoRap", "DomoCW", "DomoCCW", "TBD", "Em movimento", "TBD"] ("NomeStatus")
            w2884 = u16 3 items=["Alarme", "Atencao", "Erro", "Ocupado", "TBD", "LCB", "Trapeira", "Paravento", "DomoRap", "DomoCW", "DomoCCW", "TBD", "Em movimento", "TBD"] ("NomeStatus")
            # "MUDANÇA:\nO CW CCW comandos enviados ao controlador\nde girar e parar, estão escondidos. 26-01-2022"
            # "MUDANÇA:\nO RESET do uC CUP apaga o estado da trapeira (e paravento) o que compromote seu controle.\nNecessário implantar sensor de estado da trapeira."
            n2276 = global read "Global_Telescopio.vi" "Telescopio"() -> (w2875:bool)
            n2277 = local read "StatShutter"() -> (w2883:string)
            n2278 = local read "StatDome"() -> (w2885:string)
            n2279 = call "Bit Status CUP.vi"("NomeStatus"=w2884) -> ("StatBit"=w2881:bool)
            n2280 = Select(t=1, s=w2875, f=2) -> (s? t:f=w2873:i32)
            n2281 = event shown="[4] \"BtShutClose\": Value Change" {
              selector: _ -> [_ _ _ _ _ _ _ _]
              dyn-events: _ -> [_ _ _ _ _ _ _ _]
              timeout: 10 -> [_ _ _ _ _ _ _ _]
              tunnel: [FALSE ("NewVal") w2970 w2987 FALSE ("NewVal") FALSE ("NewVal") _ _ _] -> w2882
              tunnel: w2873 -> [_ w2969 _ _ _ _ _ _]
              event Timeout {
                n2282 = event-data() -> ()  [unwired: 1 in, 2 out]
              }
              event "BtDomeGO": Value Change {
                n2283 = event-data() -> ("NewVal"=w2971:bool)  [unwired: 1 in, 5 out]
